vi "State Machine Engine.vi"(3 "Init?":bool, 4 "Inputs":T2, 5 "Stop":bool) -> (0 "Terminated?":bool, 1 "Outputs":T3, 2 "StateData":T1)   [LabVIEW 2017]
uses:
  Controls/Outputs.ctl
  Controls/Inputs.ctl
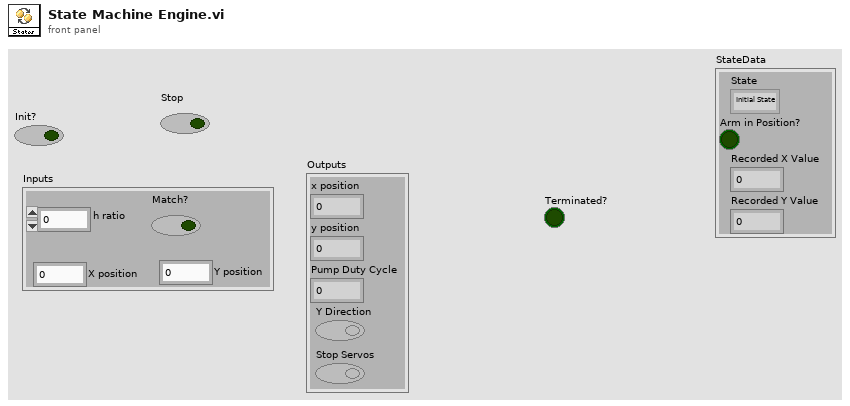
[diagram p1: front panel]
types:
  T1 = cluster{"State":enum16{"Initial State", "Pre Move", "Move Arm", "Fill Water"}, "Arm in Position?":bool, "Recorded X Value":dbl, "Recorded Y Value":dbl}
  T2 = typedef "Inputs.ctl" = cluster{"X position":dbl, "Y position":dbl, "h ratio":dbl, "Match?":bool}
  T3 = typedef "Outputs.ctl" = cluster{"x position":dbl, "y position":dbl, "Pump Duty Cycle":dbl, "Y Direction":bool, "Stop Servos":bool}
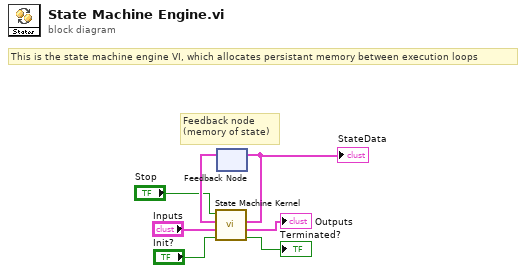
[diagram p0: block diagram]
diagram:
  # "This is the state machine engine VI, which allocates persistant memory between execution loops"
  # "Feedback node\n(memory of state)"
  n1 = feedback #1() -> (w2:T1)  [unwired: 1 in]
  n2 = call "State Machine Kernel.vi"("Init?"="Init?", "Inputs"="Inputs", "StateData"=w2, "Stop"="Stop") -> ("Terminated?"=→"Terminated?":bool, "Outputs"=→"Outputs":T3, "StateData"=w3:T1)  [unwired: 1 in]
  "StateData" <- w3
  n3 = feedback-in #1(w3) -> ()
